vi "Sapphire488GUI.vi"() -> ()   [LabVIEW 2014]
doc: "Use this template to build a user interface event handler design pattern. Use this pattern for dialog boxes and other user interfaces. You also can create and execute user-defined events that the VI can handle the same way as user interface events."
uses:
  states/488intStates.ctl
  states/488GUIStates.ctl
  <vilib>/Utility/config.llb/Read Key (String).vi
  <vilib>/Instr/_visa.llb/VISA Configure Serial Port (Instr).vi
  <vilib>/Utility/config.llb/Write Key (String).vi
  <vilib>/Utility/config.llb/NI_LVConfig.lvlib
panel:
  in  "488_High":bool
  in  "488_Low":bool
  out "Controller T":string
  out "Fault":string
  out "Diode Temp":string
  out "BasePlate T":string
  in  "SetPower [mW]":u8(slide)=20 min=20 scale=20.0..200.0
  in  "stop":bool
  out "PowesSupplyHours":string
  out "HeadHours":string
  out "Power [mW]":dbl(knob) scale=20.0..200.0
  out "?":T1
  out "Key":bool
  out "NomLP":string
  out "MaxLP":string
  out "MinLP":string
  out "Name":string
  in  "ComPort":refnum<visa-resource-name>
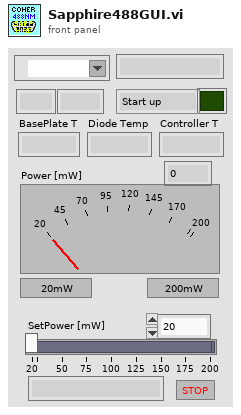
[diagram p1: front panel]
types:
  T1 = typedef "488intStates.ctl" = enum16{"Start up", "Warmup", "Standby", "Laser on", "Laser ready", "Fault"}
  T2 = typedef "488GUIStates.ctl" = enum16{"init", "startup", "idle", "stop"}
  T3 = typedef "NI_LVConfig.lvlib/Config Data RefNum.ctl" = refnum<k1>
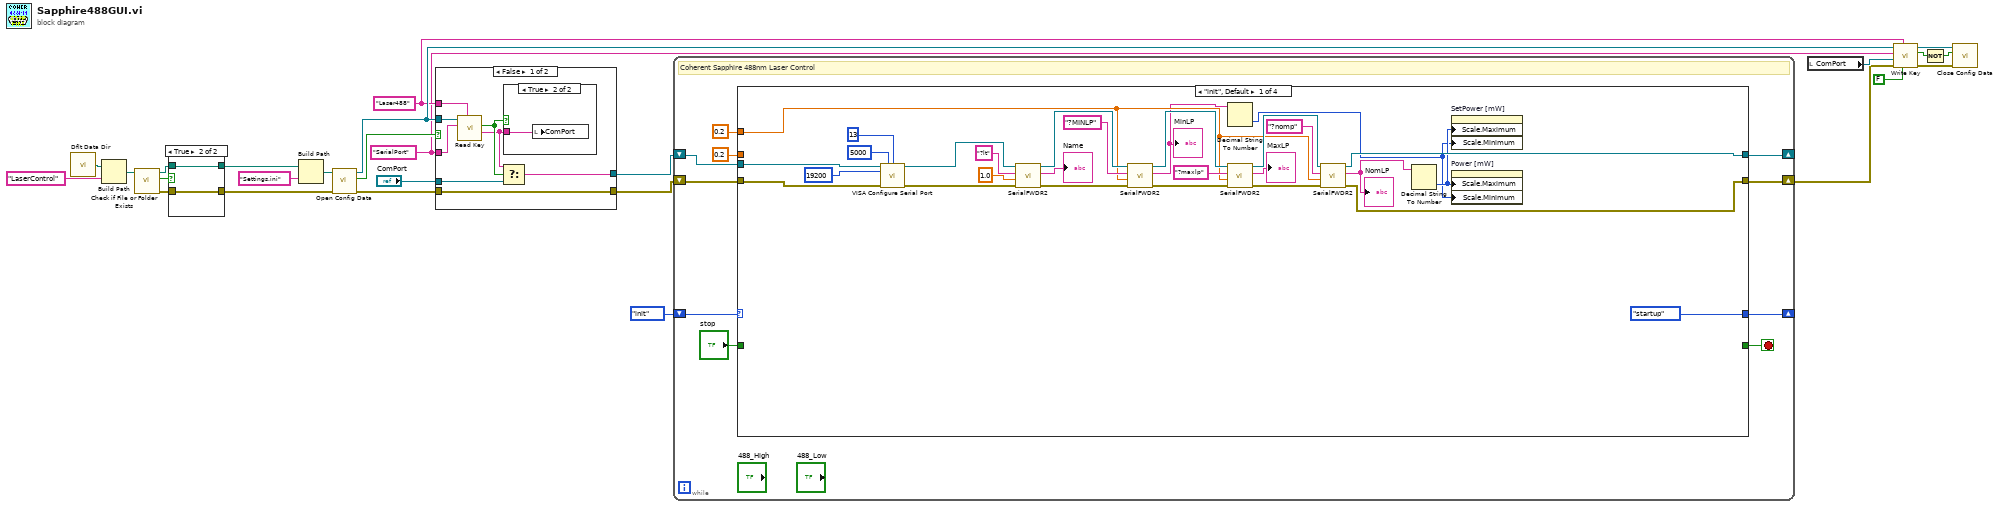
[diagram p0: block diagram]
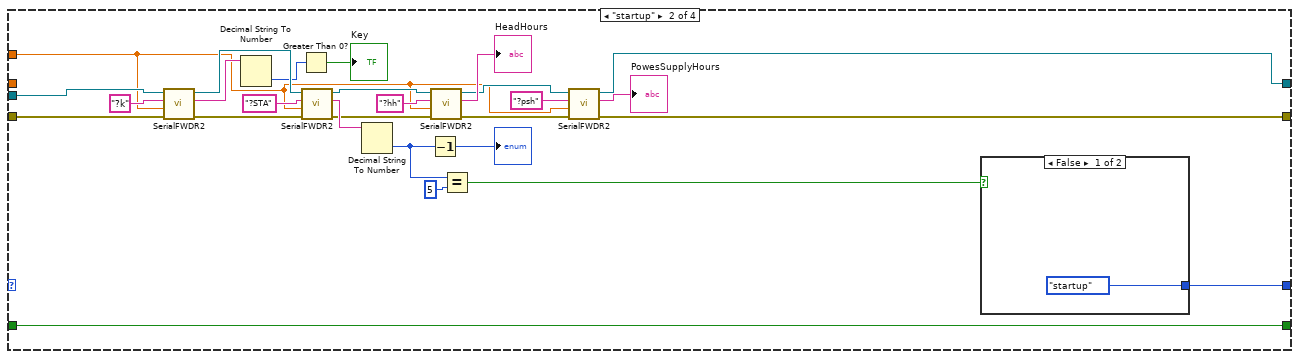
[diagram p2: hidden frame]
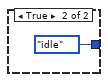
[diagram p3: hidden frame]
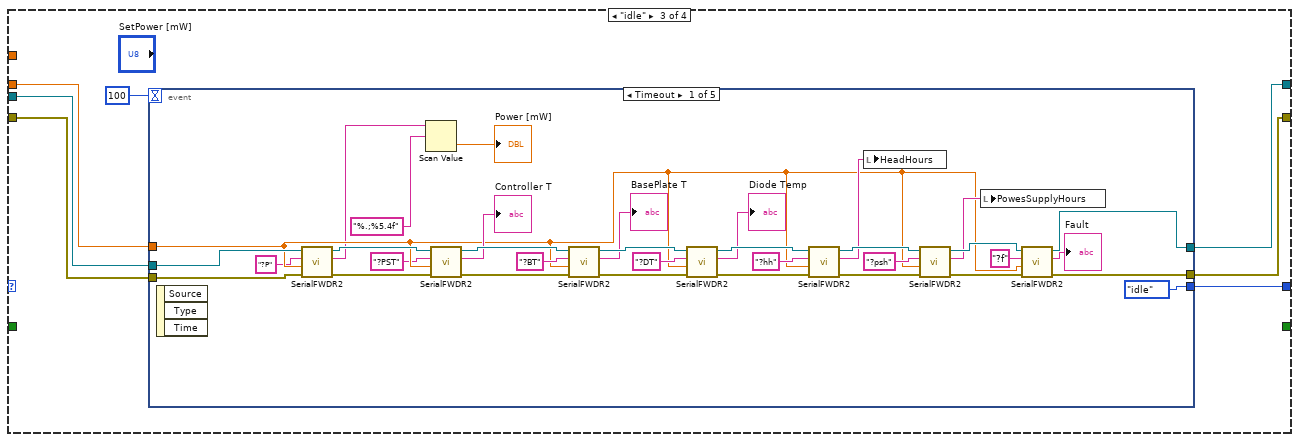
[diagram p4: hidden frame]
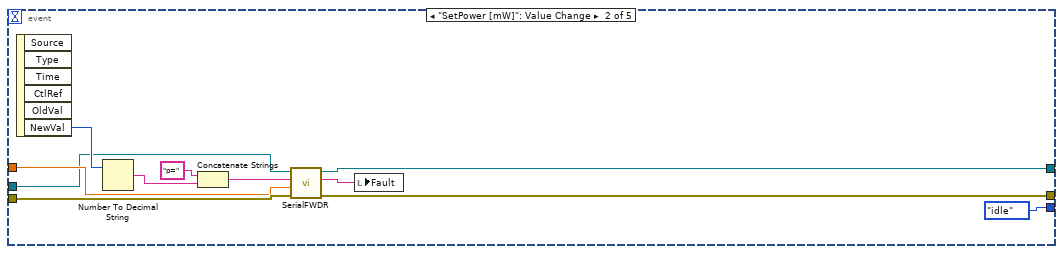
[diagram p5: hidden frame]
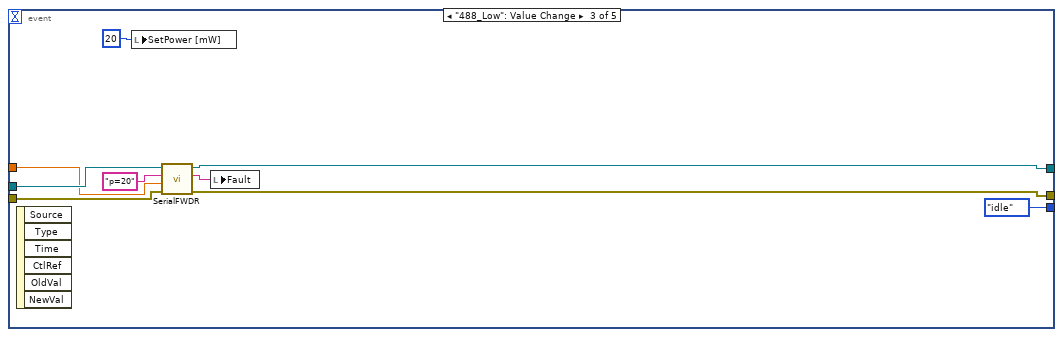
[diagram p6: hidden frame]
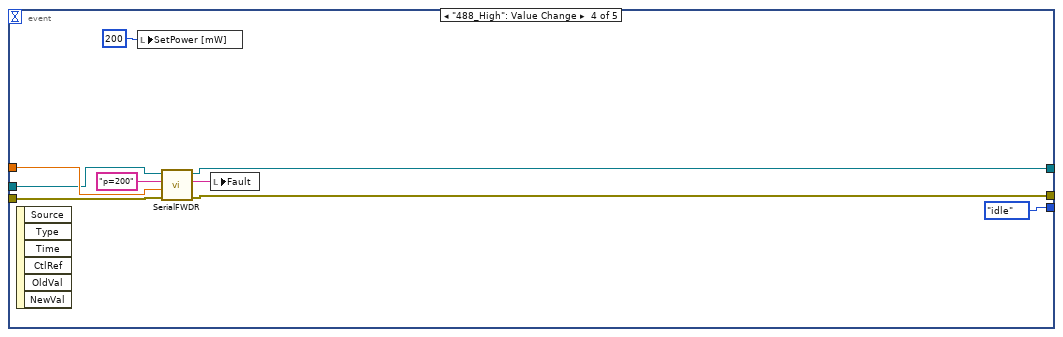
[diagram p7: hidden frame]
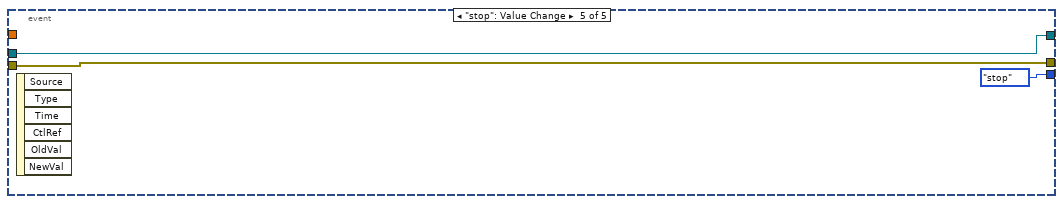
[diagram p8: hidden frame]
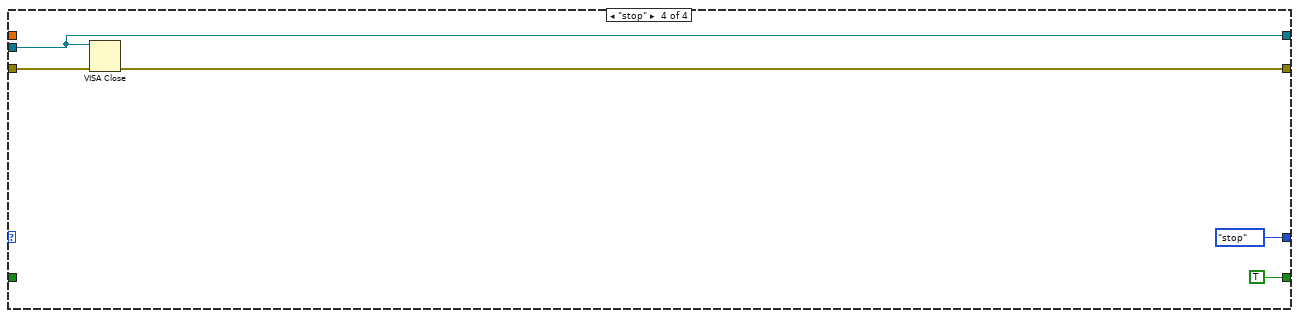
[diagram p9: hidden frame]
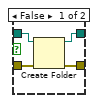
[diagram p12: hidden frame]
diagram:
  w5 = "SerialPort" ("key")
  w6 = "Laser488" ("section")
  n1 = call <vilib>:"Dflt Data Dir.vi"() -> ("App:Default Data Directory"=w22:path)
  n2 = Build Path(base path=w22, name or relative path="LaserControl") -> (appended path=w19:path)
  n3 = call <vilib>:"Check if File or Folder Exists.vi"("path"=w19) -> ("error out"=w16:errorcluster, "file or folder exists?"=w18:bool, "dup path"=w17:path)  [unwired: 8 in]
  n4 = case shown="True" w18 {
    tunnel: [w29 w32] -> w14
    tunnel: w17 -> [w30 w32]
    tunnel: w16 -> [w28 w31]
    tunnel: [w27 w31] -> w15
    frame False {
      n5 = Create Folder(path (use dialog)=w30, error in=w28) -> (created path=w29:path, error out=w27:errorcluster)  [unwired: 1 in, 1 out]
    }
    frame True {
    }
  }
  n6 = Build Path(base path=w14, name or relative path="Settings.ini") -> (appended path=w20:path)
  n7 = call <vilib>:"Open Config Data.vi"("error in (no error)"=w15, "configuration file path"=w20) -> ("error out"=w12:errorcluster, "file created?"=w9:bool, "refnum"=w10:T3)  [unwired: 7 in]
  n8 = case shown="False" w9 {
    tunnel: "ComPort" -> [w37 w43]
    tunnel: w12 -> [w36 w42]
    tunnel: w10 -> [w38 _]
    tunnel: [w36 w42] -> w3
    tunnel: [w35 w43] -> w2
    tunnel: w6 -> [w34 _]
    tunnel: w5 -> [w33 _]
    frame False {
      n9 = call-poly <vilib>:"Read Key.vi"("section"=w34, "key"=w33, "refnum"=w38) -> ("value"=w39:string, "found?"=w40:bool)  [unwired: 5 in, 2 out]
      n10 = Select(t=w39, s=w40, f=w37) -> (s? t:f=w35:string)
      n11 = case shown="True" w40 {
        tunnel: w39 -> [_ w41]
        frame False {
        }
        frame True {
          n12 = local write "ComPort"(w41) -> ()
        }
      }
    }
    frame True {
    }
  }
  n13 = while {
    shift-right: [w52] -> _
    shift-left: 488GUIStates."init" -> [w53]
    shift-right: [w49] -> _
    shift-left: w2 -> [w48]
    shift-right: [w47] -> w1
    shift-left: w3 -> [w51]
    stop <- w46 stop-if-true
    # "Coherent Sapphire 488nm Laser Control"
    n14 = case shown="\"init\", Default" w53 {
      tunnel: [488GUIStates."startup" w95 w117 488GUIStates."stop"] -> w52
      tunnel: w51 -> [w63 w108 w113 w187]
      tunnel: [w62 w86 w114 w186] -> w47
      tunnel: 0.2 ("Delay Time (s)") -> [w61 w85 _ _]
      tunnel: [w60 w88 w116 w185] -> w49
      tunnel: w48 -> [w59 w107 w115 w185]
      tunnel: [_ w82 _ TRUE] -> w46
      tunnel: "stop" -> [_ w82 _ _]
      tunnel: 0.2 ("Delay Time (s)") -> [_ _ w111 _]
      frame "init", Default {
        n15 = call-poly "VISA Configure Serial Port"("VISA resource name"=w59, "timeout (10sec)"=u32 5000, "termination char\n(0xA = '\\n' = LF)"=u8 13 ("termination char\n(0xA = '\\n' = LF)"), "baud rate (9600)"=u32 19200, "error in (no error)"=w63) -> ("VISA resource name out"=w74:refnum<visa-resource-name>, "error out"=w73:errorcluster)  [unwired: 9 in]
        n16 = call "SerialFWDR2.vi"("error in (no error)"=w73, "Delay Time (s)"=1.0, "CommandString"="?lt", "VISA Refnum in"=w74) -> ("error out"=w70:errorcluster, "trimmed string"=→"Name":string, "VISA Refnum out"=w72:refnum<visa-resource-name>)  [unwired: 5 in]
        n17 = call "SerialFWDR2.vi"("error in (no error)"=w70, "Delay Time (s)"=w61, "CommandString"="?MINLP", "VISA Refnum in"=w72) -> ("error out"=w69:errorcluster, "trimmed string"=w56:string, "VISA Refnum out"=w71:refnum<visa-resource-name>)  [unwired: 5 in]
        "MinLP" <- w56
        n18 = Decimal String To Number(string=w56) -> (number=w54:i32)  [unwired: 2 in, 1 out]
        n19 = call "SerialFWDR2.vi"("error in (no error)"=w69, "Delay Time (s)"=w61, "CommandString"="?maxlp", "VISA Refnum in"=w71) -> ("error out"=w67:errorcluster, "trimmed string"=→"MaxLP":string, "VISA Refnum out"=w68:refnum<visa-resource-name>)  [unwired: 5 in]
        n20 = call "SerialFWDR2.vi"("error in (no error)"=w67, "Delay Time (s)"=w61, "CommandString"="?nomp", "VISA Refnum in"=w68) -> ("error out"=w62:errorcluster, "trimmed string"=w58:string, "VISA Refnum out"=w60:refnum<visa-resource-name>)  [unwired: 5 in]
        "NomLP" <- w58
        n21 = Decimal String To Number(string=w58) -> (number=w55:i32)  [unwired: 2 in, 1 out]
        n22 = property on="SetPower [mW]" class="Slide (strict)"("Scale.Maximum"=w55, "Scale.Minimum"=w54) -> ()  [unwired: 2 in, 2 out]
        n23 = property on="Power [mW]" class="Knob (strict)"("Scale.Maximum"=w55, "Scale.Minimum"=w54) -> ()  [unwired: 2 in, 2 out]
      }
      frame "startup" {
        n24 = call "SerialFWDR2.vi"("error in (no error)"=w108, "Delay Time (s)"=w85, "CommandString"="?k", "VISA Refnum in"=w107) -> ("error out"=w103:errorcluster, "trimmed string"=w104:string, "VISA Refnum out"=w102:refnum<visa-resource-name>)  [unwired: 5 in]
        n25 = Decimal String To Number(string=w104) -> (number=w94:i32)  [unwired: 2 in, 1 out]
        n26 = Greater Than 0?(x=w94) -> (x > 0?=→"Key":bool)
        n27 = call "SerialFWDR2.vi"("error in (no error)"=w103, "Delay Time (s)"=w85, "CommandString"="?STA", "VISA Refnum in"=w102) -> ("error out"=w92:errorcluster, "trimmed string"=w100:string, "VISA Refnum out"=w93:refnum<visa-resource-name>)  [unwired: 5 in]
        n28 = Decimal String To Number(string=w100) -> (number=w97:i32)  [unwired: 2 in, 1 out]
        n29 = Decrement(x=w97) -> (x-1=→"?":i32)
        n30 = call "SerialFWDR2.vi"("error in (no error)"=w92, "Delay Time (s)"=w85, "CommandString"="?hh", "VISA Refnum in"=w93) -> ("error out"=w87:errorcluster, "trimmed string"=→"HeadHours":string, "VISA Refnum out"=w89:refnum<visa-resource-name>)  [unwired: 5 in]
        n31 = Equal?(x=w97, y=5) -> (x = y?=w96:bool)
        n32 = call "SerialFWDR2.vi"("error in (no error)"=w87, "Delay Time (s)"=w85, "CommandString"="?psh", "VISA Refnum in"=w89) -> ("error out"=w86:errorcluster, "trimmed string"=→"PowesSupplyHours":string, "VISA Refnum out"=w88:refnum<visa-resource-name>)  [unwired: 5 in]
        n33 = case shown="False" w96 {
          tunnel: [488GUIStates."startup" 488GUIStates."idle"] -> w95
          frame False {
          }
          frame True {
          }
        }
      }
      frame "idle" {
        n34 = event shown="[0] Timeout" {
          selector: _ -> [_ _ _ _ _]
          dyn-events: _ -> [_ _ _ _ _]
          timeout: 100 -> [_ _ _ _ _]
          tunnel: [488GUIStates."idle" 488GUIStates."idle" 488GUIStates."idle" 488GUIStates."idle" 488GUIStates."stop"] -> w117
          tunnel: [w118 w153 w168 w176 w182] -> w116
          tunnel: w115 -> [w127 w154 w167 w173 w182]
          tunnel: [w119 w157 w169 w178 w181] -> w114
          tunnel: w113 -> [w126 w158 w170 w179 w181]
          tunnel: w111 -> [w125 w156 w164 w174 _]
          event Timeout {
            n35 = event-data() -> ()  [unwired: 1 in, 3 out]
            n36 = call "SerialFWDR2.vi"("error in (no error)"=w126, "Delay Time (s)"=w125, "CommandString"="?P", "VISA Refnum in"=w127) -> ("error out"=w128:errorcluster, "trimmed string"=w121:string, "VISA Refnum out"=w129:refnum<visa-resource-name>)  [unwired: 5 in]
            n37 = Scan Value(string=w121, format string="%.;%5.4f") -> (value=→"Power [mW]":dbl)  [unwired: 1 in, 1 out]
            n38 = call "SerialFWDR2.vi"("error in (no error)"=w128, "Delay Time (s)"=w125, "CommandString"="?PST", "VISA Refnum in"=w129) -> ("error out"=w131:errorcluster, "trimmed string"=→"Controller T":string, "VISA Refnum out"=w132:refnum<visa-resource-name>)  [unwired: 5 in]
            n39 = call "SerialFWDR2.vi"("error in (no error)"=w131, "Delay Time (s)"=w125, "CommandString"="?BT", "VISA Refnum in"=w132) -> ("error out"=w146:errorcluster, "trimmed string"=→"BasePlate T":string, "VISA Refnum out"=w150:refnum<visa-resource-name>)  [unwired: 5 in]
            n40 = call "SerialFWDR2.vi"("error in (no error)"=w146, "Delay Time (s)"=w125, "CommandString"="?DT", "VISA Refnum in"=w150) -> ("error out"=w145:errorcluster, "trimmed string"=→"Diode Temp":string, "VISA Refnum out"=w149:refnum<visa-resource-name>)  [unwired: 5 in]
            n41 = call "SerialFWDR2.vi"("error in (no error)"=w145, "Delay Time (s)"=w125, "CommandString"="?hh", "VISA Refnum in"=w149) -> ("error out"=w144:errorcluster, "trimmed string"=w137:string, "VISA Refnum out"=w148:refnum<visa-resource-name>)  [unwired: 5 in]
            n42 = local write "HeadHours"(w137) -> ()
            n43 = call "SerialFWDR2.vi"("error in (no error)"=w144, "Delay Time (s)"=w125, "CommandString"="?psh", "VISA Refnum in"=w148) -> ("error out"=w143:errorcluster, "trimmed string"=w135:string, "VISA Refnum out"=w147:refnum<visa-resource-name>)  [unwired: 5 in]
            n44 = local write "PowesSupplyHours"(w135) -> ()
            n45 = call "SerialFWDR2.vi"("error in (no error)"=w143, "Delay Time (s)"=w125, "CommandString"="?f", "VISA Refnum in"=w147) -> ("error out"=w119:errorcluster, "trimmed string"=→"Fault":string, "VISA Refnum out"=w118:refnum<visa-resource-name>)  [unwired: 5 in]
          }
          event "SetPower [mW]": Value Change {
            n46 = event-data() -> ("NewVal"=w161:u8)  [unwired: 1 in, 5 out]
            n47 = Number To Decimal String(number=w161) -> (decimal integer string=w160:string)  [unwired: 1 in]
            n48 = Concatenate Strings("p=", w160) -> (w155:string)
            n49 = call "SerialFWDR.vi"("error in (no error)"=w158, "Delay Time (s)"=w156, "CommandString"=w155, "VISA Refnum in"=w154) -> ("error out"=w157:errorcluster, "trimmed string"=w152:string, "VISA Refnum out"=w153:refnum<visa-resource-name>)  [unwired: 5 in]
            n50 = local write "Fault"(w152) -> ()
          }
          event "488_Low": Value Change {
            n51 = event-data() -> ()  [unwired: 1 in, 6 out]
            n52 = local write "SetPower [mW]"(u8 20 ("SetPower [mW]")) -> ()
            n53 = call "SerialFWDR.vi"("error in (no error)"=w170, "Delay Time (s)"=w164, "CommandString"="p=20", "VISA Refnum in"=w167) -> ("error out"=w169:errorcluster, "trimmed string"=w166:string, "VISA Refnum out"=w168:refnum<visa-resource-name>)  [unwired: 5 in]
            n54 = local write "Fault"(w166) -> ()
          }
          event "488_High": Value Change {
            n55 = event-data() -> ()  [unwired: 1 in, 6 out]
            n56 = local write "SetPower [mW]"(u8 200 ("SetPower [mW]")) -> ()
            n57 = call "SerialFWDR.vi"("error in (no error)"=w179, "Delay Time (s)"=w174, "CommandString"="p=200", "VISA Refnum in"=w173) -> ("error out"=w178:errorcluster, "trimmed string"=w177:string, "VISA Refnum out"=w176:refnum<visa-resource-name>)  [unwired: 5 in]
            n58 = local write "Fault"(w177) -> ()
          }
          event "stop": Value Change {
            n59 = event-data() -> ()  [unwired: 1 in, 6 out]
          }
        }
      }
      frame "stop" {
        n60 = VISA Close(VISA resource name=w185, error in (no error)=w187) -> (error out=w186:errorcluster)
      }
    }
  }
  n61 = local read "ComPort"() -> (w25:refnum<visa-resource-name>)
  n62 = call-poly <vilib>:"Write Key.vi"("write raw string? (F)"=FALSE, "section"=w6, "error in (no error)"=w1, "value"=w25, "key"=w5, "refnum"=w10) -> ("error out"=w23:errorcluster, "found?"=w8:bool, "refnum out"=w24:T3)  [unwired: 3 in]
  n63 = Not(x=w8) -> (.not. x?=w7:bool)
  n64 = call <vilib>:"Close Config Data.vi"("error in (no error)"=w23, "write file if changed (T)"=w7, "refnum"=w24) -> ()  [unwired: 7 in, 2 out]
